vi "MCA_slave.vi"() -> (0 "波形图":i32[](graph))   [LabVIEW 2014]
panel:
  out "和":i32
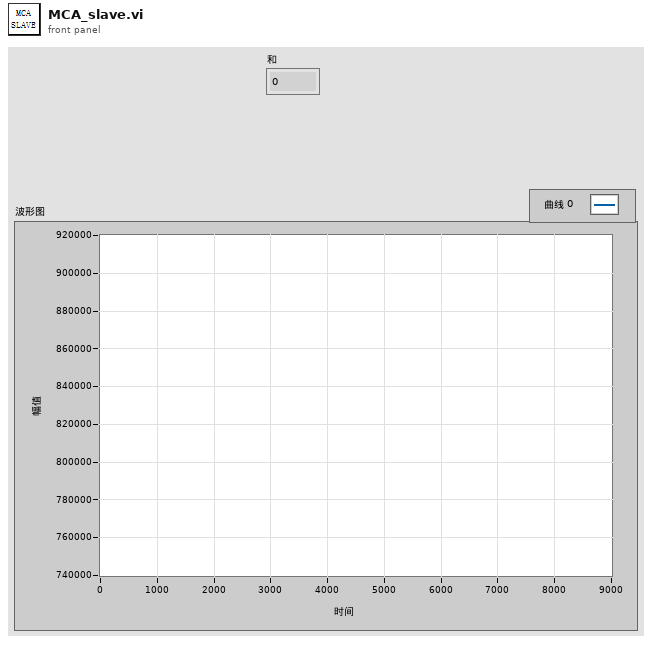
[diagram p1: front panel]
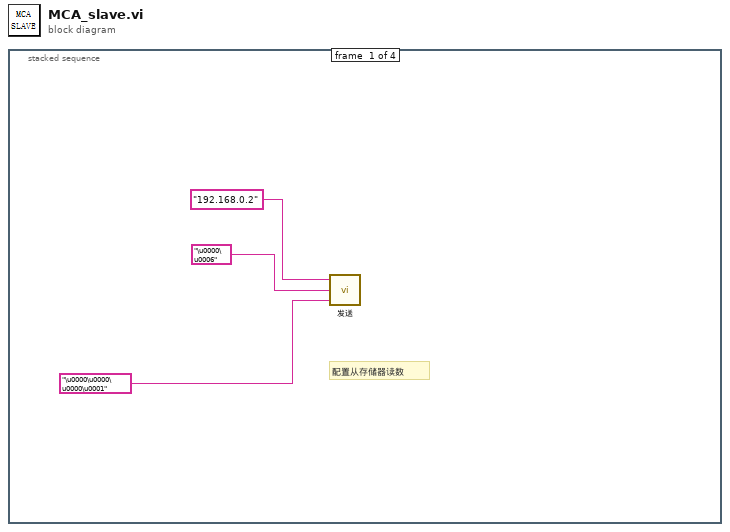
[diagram p0: block diagram]
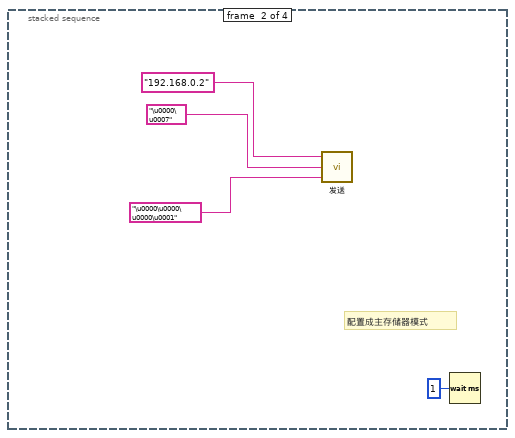
[diagram p2: hidden frame]
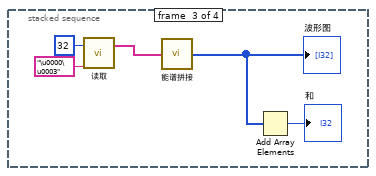
[diagram p3: hidden frame]
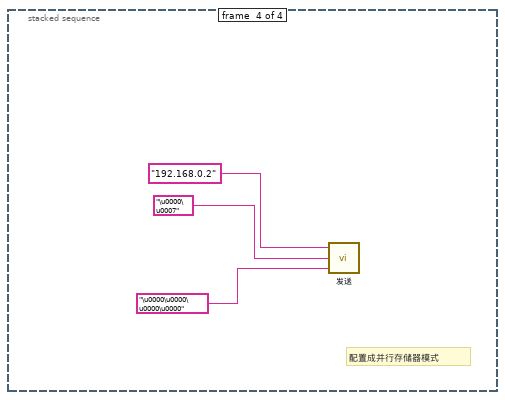
[diagram p4: hidden frame]
diagram:
  n1 = stacked-sequence {
    frame #0 {
      # "配置从存储器读数"
      n2 = call "发送.vi"("数据（32bit）"="\u0000\u0000\u0000\u0001", "命令(16bit)"="\u0000\u0006", "目标IP"="192.168.0.2") -> ()  [unwired: 1 out]
    }
    frame #1 {
      # "配置成主存储器模式"
      n3 = call "发送.vi"("数据（32bit）"="\u0000\u0000\u0000\u0001", "命令(16bit)"="\u0000\u0007", "目标IP"="192.168.0.2") -> ()  [unwired: 1 out]
      n4 = Wait (ms)(milliseconds to wait=u32 1 ("等待时间（毫秒）")) -> ()  [unwired: 1 out]
    }
    frame #2 {
      n5 = call "读取.vi"("命令"="\u0000\u0003", "帧数"=32) -> ("数组"=w9:string[])  [unwired: 1 out]
      n6 = call "能谱拼接.vi"("数组"=w9) -> ("拼接数组"=w8:i32[])
      "波形图" <- w8
      n7 = Add Array Elements(numeric array=w8) -> (sum=→"和":i32)
    }
    frame #3 {
      # "配置成并行存储器模式"
      n8 = call "发送.vi"("数据（32bit）"="\u0000\u0000\u0000\u0000", "命令(16bit)"="\u0000\u0007", "目标IP"="192.168.0.2") -> ()  [unwired: 1 out]
    }
  }
